vi "Cmd_G_OK.vi"(0 "reference":refnum<visa-resource-name>, 7 "Command String":string) -> (4 "reference dup":refnum<visa-resource-name>, 8 "OK Done":bool, 15 "error OUT":errorcluster)   [LabVIEW 2011]
panel:
  # "Port Number 0=COM1"
  # "Send 'Command String', receive 'OK', send 'G Command' and receive 'OK'."
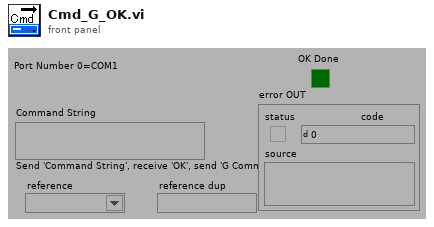
[diagram p1: front panel]
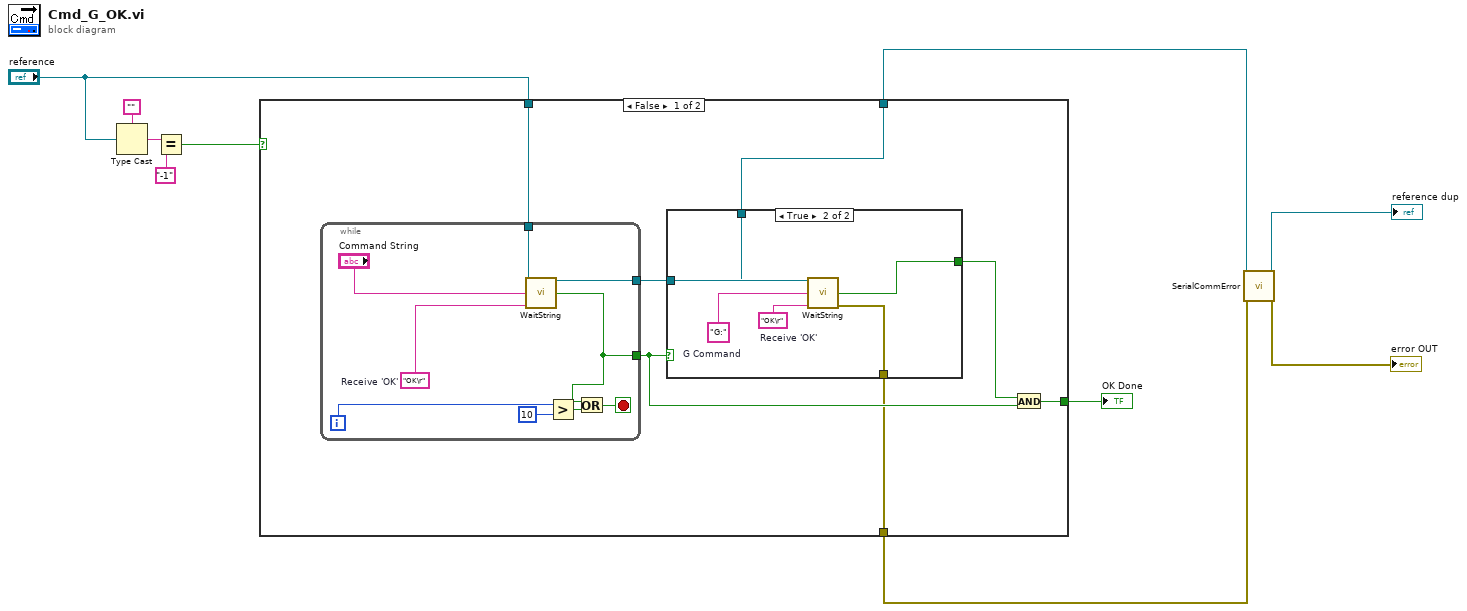
[diagram p0: block diagram]
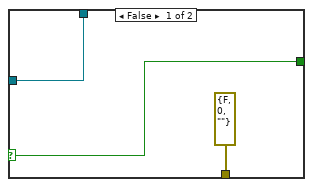
[diagram p2: hidden frame]
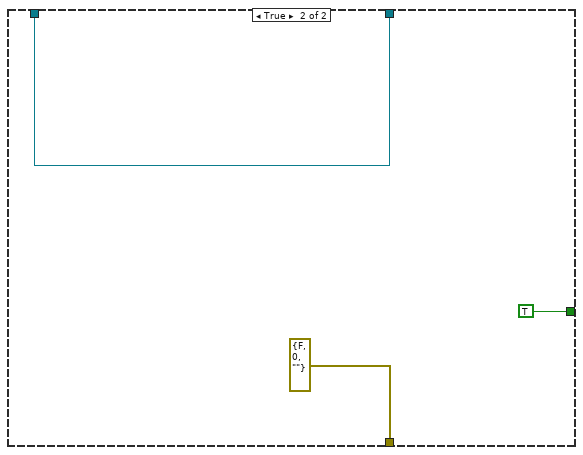
[diagram p3: hidden frame]
diagram:
  n1 = Type Cast(type="", x="reference") -> (*(type *) &x=w8:string)
  n2 = Equal?(x=w8, y="-1") -> (x = y?=w5:bool)
  n3 = case shown="False" w5 {
    tunnel: [w17 TRUE] -> w10
    tunnel: "reference" -> [w13 w37]
    tunnel: [w12 w37] -> w3
    tunnel: [w11 errorcluster {"status"=FALSE, "code"=0, "source"=""} ("error out")] -> w4
    frame False {
      n4 = while {
        tunnel: [w21] -> w15
        tunnel: w13 -> [w20]
        tunnel: [w19] -> w14
        i -> [w24]
        stop <- w22 stop-if-true
        w26 = "OK\r"  # Receive 'OK'
        n5 = call "WaitString.vi"("reference"=w20, "String to Send"="Command String", "String to Receive"=w26) -> ("reference dup"=w19:refnum<visa-resource-name>, "OK Done"=w21:bool)  [unwired: 10 in, 1 out]
        n6 = Greater?(x=w24, y=10) -> (0:w25:bool)
        n7 = Or(x=w21, y=w25) -> (x .or. y?=w22:bool)
      }
      n8 = case shown="True" w15 {
        selector: w15 -> [w29 _]
        tunnel: [w29 w33] -> w16
        tunnel: w14 -> [w28 w32]
        tunnel: [w28 w31] -> w12
        tunnel: [errorcluster {"status"=FALSE, "code"=0, "source"=""} ("error out") w30] -> w11
        frame False {
        }
        frame True {
          w34 = "OK\r"  # Receive 'OK'
          w35 = "G:"  # G Command
          n9 = call "WaitString.vi"("reference"=w32, "String to Send"=w35, "String to Receive"=w34) -> ("reference dup"=w31:refnum<visa-resource-name>, "OK Done"=w33:bool, "error out"=w30:errorcluster)  [unwired: 10 in]
        }
      }
      n10 = And(x=w16, y=w15) -> (x .and. y?=w17:bool)
    }
    frame True {
    }
  }
  "OK Done" <- w10
  n11 = call "SerialCommError.vi"("VISA IN"=w3, "error IN"=w4) -> ("VISA OUT"=→"reference dup":refnum<visa-resource-name>, "error OUT"=→"error OUT":errorcluster)  [unwired: 11 in, 1 out]
